vi "Get Alarm Control Refnum.vi"(8 "error in (no error)":errorcluster, 9 "Active Alarm?":bool, 10 "Subsystem URL":refnum<k21>, 11 "Reference URL Map In":variant) -> (0 "error out":errorcluster, 1 "Found?":bool, 2 "Control Refnum":refnum<vi>, 3 "Reference URL Map Out":variant)   [LabVIEW 2024]
doc: "Gets the control refnum from the map."
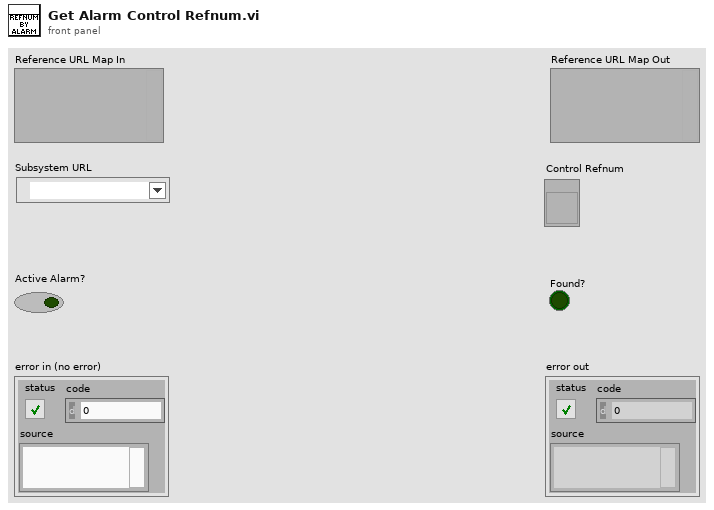
[diagram p1: front panel]
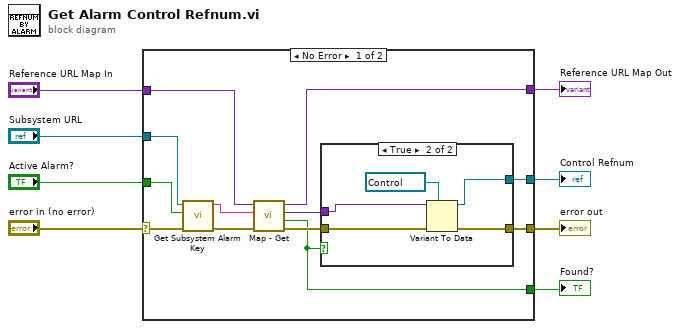
[diagram p0: block diagram]
diagram:
  n1 = case shown="No Error" "error in (no error)" {
    selector: "error in (no error)" -> [w18 w28]
    tunnel: [w12 w28] -> w7
    tunnel: "Reference URL Map In" -> [w17 w27]
    tunnel: [w16 w27] -> w5
    tunnel: "Active Alarm?" -> [w15 _]
    tunnel: "Subsystem URL" -> [w14 _]
    tunnel: [w10 _] -> w2
    tunnel: [w9 _] -> w1
    frame No Error {
      n2 = call "Get Subsystem Alarm Key.vi"("error in (no error)"=w18, "Active Alarm?"=w15, "Subsystem URL"=w14) -> ("error out"=w20:errorcluster, "Subsystem Alarm Key"=w19:string)  [unwired: 7 in]
      n3 = call "Map - Get.vi"("error in (no error)"=w20, "Key"=w19, "Map In"=w17) -> ("error out"=w13:errorcluster, "Found?"=w10:bool, "Value"=w11:variant, "Map Out"=w16:variant)  [unwired: 5 in]
      n4 = case shown="True" w10 {
        tunnel: w13 -> [w21 w25]
        tunnel: [w21 w24] -> w12
        tunnel: w11 -> [_ w23]
        tunnel: [_ w22] -> w9
        frame False {
        }
        frame True {
          n5 = Variant To Data(error in=w25, type=refnum<vi> refnum ("Ctl Refnum"), Variant=w23) -> (data=w22:refnum<vi>, error out=w24:errorcluster)
        }
      }
    }
    frame Error {
    }
  }
  "error out" <- w7
  "Reference URL Map Out" <- w5
  "Control Refnum" <- w1
  "Found?" <- w2
